vi "Write Display Message.vi"(0 "VISA resource name":refnum<visa-resource-name>, 1 "Message (\"\")":string, 5 "Message Number (1)":i32=1 min=1 max=100 step=1, 7 "Destination (0 : Specified Group)":i32(ring) items=["Specified Group", "All Groups"], 9 "Group Number (1)":string="1", 11 "error in (no error)":errorcluster) -> (4 "VISA resource name out":refnum<visa-resource-name>, 15 "error out":errorcluster)   [LabVIEW 2020, in "Yokogawa GX Series.lvlib"]
doc: "Writes the message.\nThis command displays the message to the screen and writes the message into the display data and event data."
uses:
  <instrlib>/Yokogawa GX Series/Yokogawa GX Series.lvlib
panel:
  in  "Batch Group Number  (0: OFF)":i32(ring) items=["OFF", "1", "2", "3", "4", "5", "6", "7", "8", "9", "10", "11", "12"]
  in  "Action Type (0: Preset Message)":i32(ring) items=["Preset", "Free"]
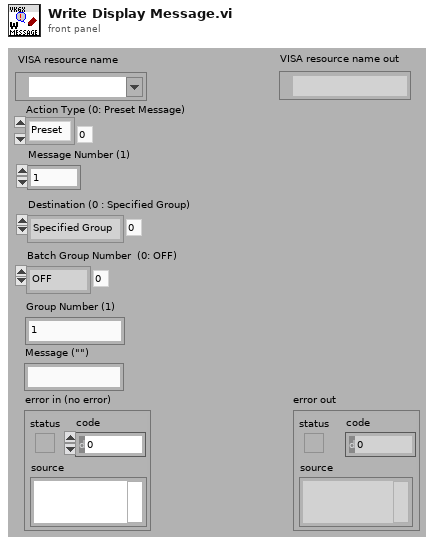
[diagram p1: front panel]
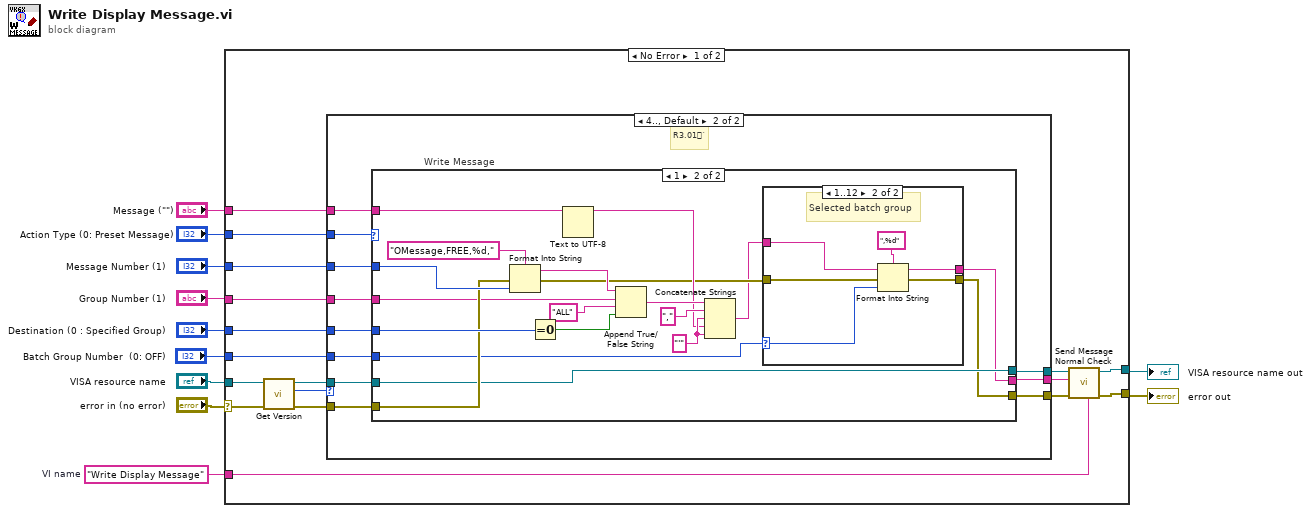
[diagram p0: block diagram]
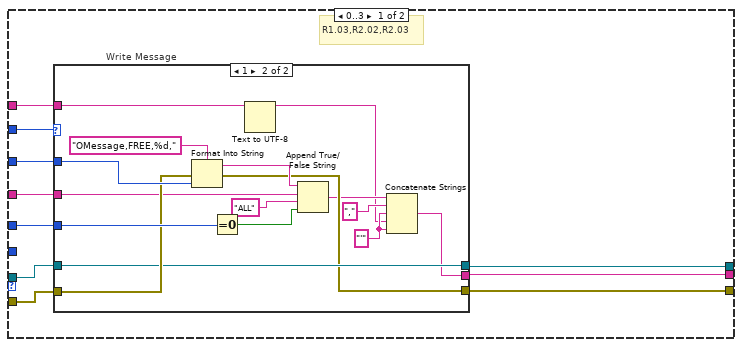
[diagram p2: hidden frame]
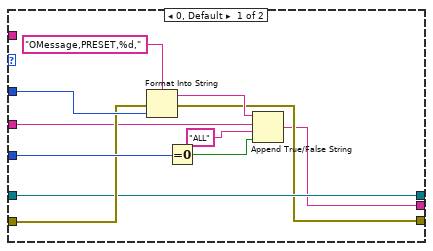
[diagram p3: hidden frame]
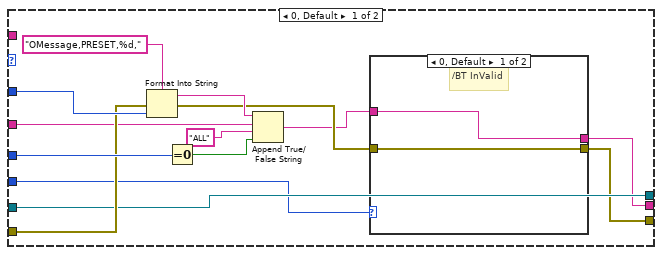
[diagram p4: hidden frame]
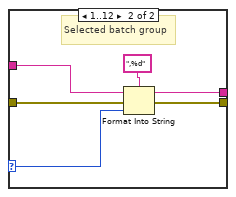
[diagram p5: hidden frame]
diagram:
  w9 = "Write Display Message"  # VI name
  n1 = case shown="No Error" "error in (no error)" {
    selector: "error in (no error)" -> [w18 w126]
    tunnel: "Message Number (1)" -> [w28 _]
    tunnel: "VISA resource name" -> [w19 w127]
    tunnel: w9 -> [w23 _]
    tunnel: [w25 w127] -> w8
    tunnel: "Destination (0 : Specified Group)" -> [w27 _]
    tunnel: "Group Number (1)" -> [w26 _]
    tunnel: [w24 w126] -> w5
    tunnel: "Action Type (0: Preset Message)" -> [w22 _]
    tunnel: "Message (\"\")" -> [w20 _]
    tunnel: "Batch Group Number  (0: OFF)" -> [w12 _]
    frame No Error {
      n2 = call <instrlib>:"Get Version.vi"("error in (no error)"=w18, "VISA resource name"=w19) -> ("error out"=w16:errorcluster, "Version"=w13:i32, "VISA resource name out"=w17:refnum<visa-resource-name>)  [unwired: 7 in]
      n3 = case shown="4.., Default" w13 {
        tunnel: w28 -> [w38 w76]
        tunnel: w27 -> [w37 w75]
        tunnel: w26 -> [w36 w74]
        tunnel: w22 -> [w35 w73]
        tunnel: [w34 w72] -> w21
        tunnel: [w29 w67] -> w15
        tunnel: [w33 w71] -> w14
        tunnel: w20 -> [w32 w70]
        tunnel: w17 -> [w31 w69]
        tunnel: w16 -> [w30 w68]
        tunnel: w12 -> [_ w66]
        frame 0..3 {
          # "Write Message"
          # "R1.03,R2.02,R2.03"
          n4 = case shown="1" w35 {
            tunnel: w38 -> [w49 w65]
            tunnel: w31 -> [w41 w57]
            tunnel: w37 -> [w48 w64]
            tunnel: w36 -> [w43 w59]
            tunnel: w30 -> [w45 w61]
            tunnel: [w41 w57] -> w29
            tunnel: [w40 w56] -> w34
            tunnel: [w39 w53] -> w33
            tunnel: w32 -> [_ w51]
            frame 0, Default {
              n5 = Format Into String(format string="OMessage,PRESET,%d,", error in=w45, w49) -> (resulting string=w47:string, error out=w40:errorcluster)  [unwired: 1 in]
              n6 = Equal To 0?(x=w48) -> (x = 0?=w46:bool)
              n7 = Append True/False String(1:w46, 2:"ALL", 3:w43, 4:w47) -> (0:w39:string)
            }
            frame 1 {
              w52 = "'"
              n8 = Format Into String(format string="OMessage,FREE,%d,", error in=w61, w65) -> (resulting string=w63:string, error out=w56:errorcluster)  [unwired: 1 in]
              n9 = Equal To 0?(x=w64) -> (x = 0?=w62:bool)
              n10 = Text to UTF-8(11:w51) -> (3:w50:string)  [unwired: 2 in, 1 out]
              n11 = Append True/False String(1:w62, 2:"ALL", 3:w59, 4:w63) -> (0:w55:string)
              n12 = Concatenate Strings(w55, ",", w52, w50, w52) -> (w53:string)
            }
          }
        }
        frame 4.., Default {
          # "Write Message"
          # "R3.01`"
          n13 = case shown="1" w73 {
            tunnel: w76 -> [w90 w117]
            tunnel: w69 -> [w82 w109]
            tunnel: w75 -> [w89 w116]
            tunnel: w74 -> [w84 w111]
            tunnel: w68 -> [w86 w113]
            tunnel: [w82 w109] -> w67
            tunnel: [w78 w102] -> w72
            tunnel: [w79 w101] -> w71
            tunnel: w70 -> [_ w105]
            tunnel: w66 -> [w77 w99]
            frame 0, Default {
              n14 = Format Into String(format string="OMessage,PRESET,%d,", error in=w86, w90) -> (resulting string=w88:string, error out=w81:errorcluster)  [unwired: 1 in]
              n15 = Equal To 0?(x=w89) -> (x = 0?=w87:bool)
              n16 = Append True/False String(1:w87, 2:"ALL", 3:w84, 4:w88) -> (0:w80:string)
              n17 = case shown="0, Default" w77 {
                selector: w77 -> [_ w93]
                tunnel: w80 -> [w92 w97]
                tunnel: w81 -> [w91 w96]
                tunnel: [w91 w95] -> w78
                tunnel: [w92 w94] -> w79
                frame 0, Default {
                  # "/BT InValid"
                }
                frame 1..12 {
                  # "Selected batch group"
                  n18 = Format Into String(format string=",%d", initial string=w97, error in=w96, w93) -> (resulting string=w94:string, error out=w95:errorcluster)
                }
              }
            }
            frame 1 {
              w106 = "'"
              n19 = Format Into String(format string="OMessage,FREE,%d,", error in=w113, w117) -> (resulting string=w115:string, error out=w103:errorcluster)  [unwired: 1 in]
              n20 = Equal To 0?(x=w116) -> (x = 0?=w114:bool)
              n21 = Text to UTF-8(11:w105) -> (3:w104:string)  [unwired: 2 in, 1 out]
              n22 = Append True/False String(1:w114, 2:"ALL", 3:w111, 4:w115) -> (0:w108:string)
              n23 = Concatenate Strings(w108, ",", w106, w104, w106) -> (w100:string)
              n24 = case shown="1..12" w99 {
                selector: w99 -> [_ w120]
                tunnel: w100 -> [w119 w124]
                tunnel: w103 -> [w118 w123]
                tunnel: [w118 w122] -> w102
                tunnel: [w119 w121] -> w101
                frame 0, Default {
                  # "/BT InValid"
                }
                frame 1..12 {
                  # "Selected batch group"
                  n25 = Format Into String(format string=",%d", initial string=w124, error in=w123, w120) -> (resulting string=w121:string, error out=w122:errorcluster)
                }
              }
            }
          }
        }
      }
      n26 = call <instrlib>:"Send Message Normal Check.vi"("Source (\"\")"=w23, "error in (no error)"=w21, "Send Message (\"\")"=w14, "VISA resource name"=w15) -> ("error out"=w24:errorcluster, "VISA resource name out"=w25:refnum<visa-resource-name>)  [unwired: 2 in, 4 out]
    }
    frame Error {
    }
  }
  "error out" <- w5
  "VISA resource name out" <- w8
